vi "Server.vi"() -> ()   [LabVIEW 2024]
uses:
  <vilib>/Utility/file.llb/Write Delimited Spreadsheet (string).vi
panel:
  out "Humidity":dbl(graph)
  out "Temperature":dbl(graph)
  out "TIME":string
  out "DATE":string
  out "Particles Per Million":dbl(graph)
  in  "STOP":bool
  out "CO2 PPM":dbl(slide) scale=0.0..1000.0
  out "Humidity":dbl(slide) scale=0.0..100.0
  out "Temperature":dbl(slide) scale=0.0..50.0
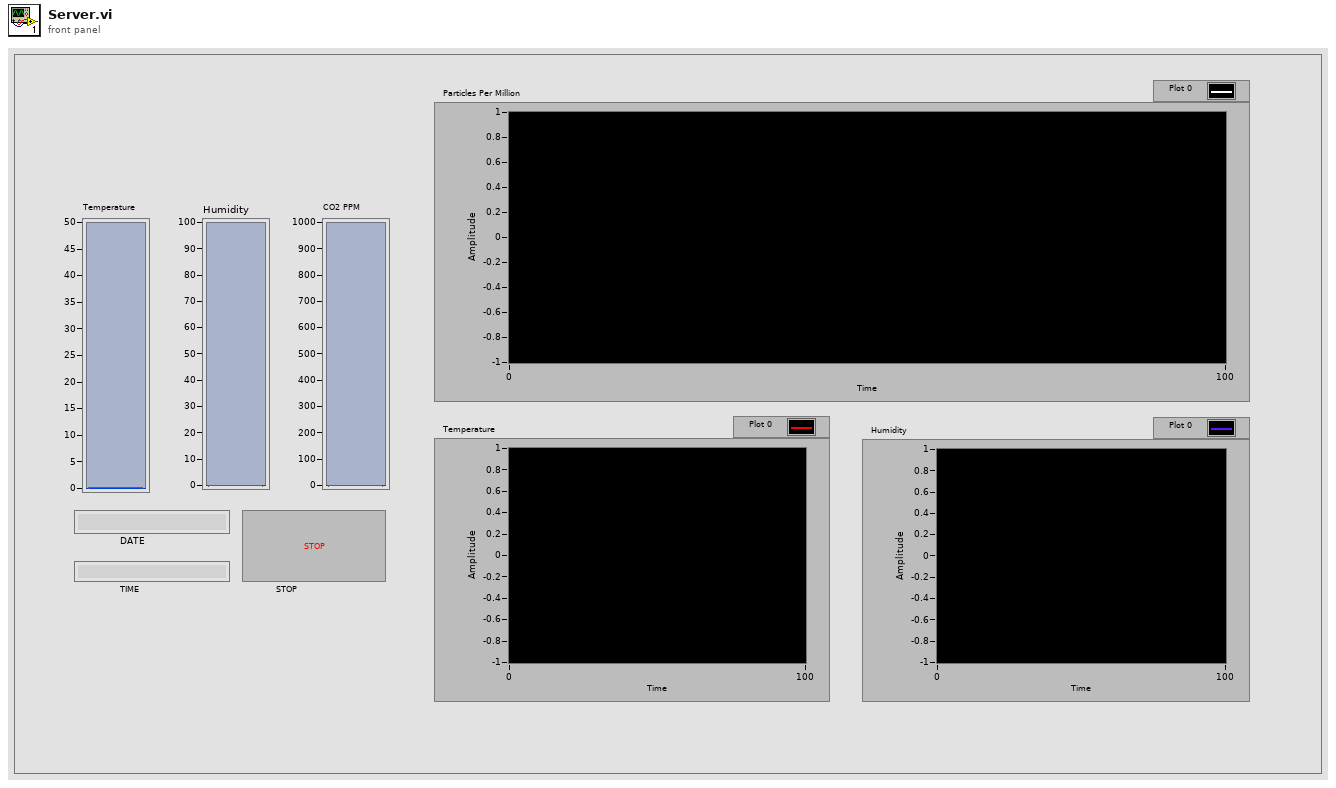
[diagram p1: front panel]
types:
  T1 = enum16{"Standard", "Buffered", "CRLF", "Immediate"}
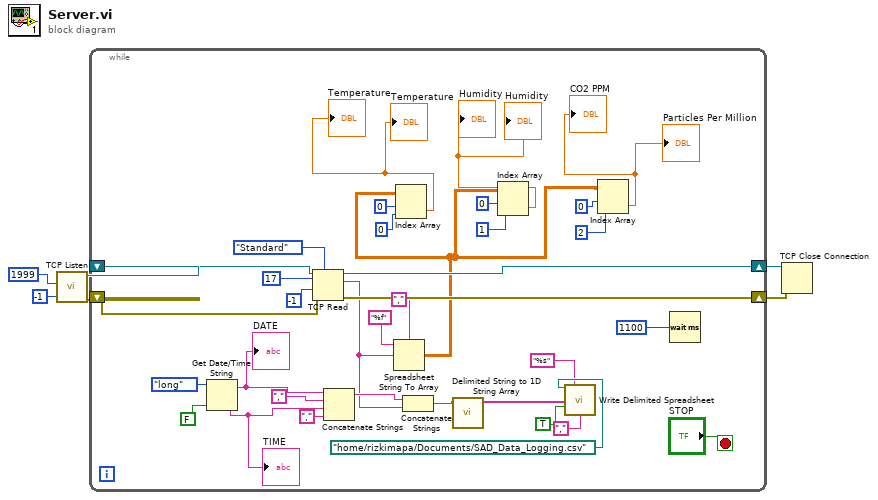
[diagram p0: block diagram]
diagram:
  n1 = call <vilib>:"TCP Listen.vi"("timeout ms (wait forever: -1)"=-1, "port"=u16 1999) -> ("error out"=w4:errorcluster, "connection ID"=w6:refnum<k5>)  [unwired: 5 in, 3 out]
  n2 = while {
    shift-right: [w38] -> w5
    shift-left: w6 -> [w41]
    shift-right: [w37] -> w3
    shift-left: w4 -> [w40]
    stop <- "STOP" stop-if-true
    n3 = Get Date/Time String(date format (0)=enum16{"short", "long", "abbreviated"}."long", want seconds? (F)=FALSE) -> (date string=w12:string, time string=w11:string)  [unwired: 1 in]
    "DATE" <- w12
    "TIME" <- w11
    n4 = TCP Read(connection ID=w41, bytes to read=17, error in (no error)=w40, 7:T1."Standard" ("mode (standard)"), 9:-1 ("timeout ms (25000)")) -> (connection ID out=w38:refnum<k5>, data out=w21:string, error out=w37:errorcluster)
    n5 = Concatenate Strings(w12, "," ("string"), w11, "," ("string")) -> (w22:string)
    n6 = Spreadsheet String To Array(delimiter (Tab)=",", format string="%f", spreadsheet string=w21) -> (array=w10:dbl[][])  [unwired: 1 in]
    n7 = Index Array(array=w10, index (row)=0, index (col)=0 ("disabled index (col)")) -> (element=→"Temperature" →"Temperature":dbl)
    n8 = Concatenate Strings(w22, w21) -> (w14:string)
    n9 = call <vilib>:"Delimited String to 1D String Array.vi"("delimited string"=w14) -> ("string array"=w13:string[])  [unwired: 10 in]
    n10 = Index Array(array=w10, index (row)=0, index (col)=1 ("disabled index (col)")) -> (element=→"Humidity" →"Humidity":dbl)
    n11 = call-poly <vilib>:"Write Delimited Spreadsheet.vi"("file path (dialog if empty)"=path "/home/rizkimapa/Documents/SAD_Data_Logging.csv", "format (%s)"="%s" ("format (%.3f)"), "1D data"=w13, "append to file? (new file:F)"=TRUE, "delimiter (\\t)"="," ("delimiter (\\t)")) -> ()  [unwired: 9 in, 2 out]
    n12 = Index Array(array=w10, index (row)=0, index (col)=2 ("disabled index (col)")) -> (element=→"CO2 PPM" →"Particles Per Million":dbl)
    n13 = Wait (ms)(milliseconds to wait=u32 1100) -> ()  [unwired: 1 out]
  }
  n14 = TCP Close Connection(connection ID=w5, error in (no error)=w3) -> ()  [unwired: 1 in, 2 out]
